vi "1st CMD Operations.vi"(8 "error in (no error)":errorcluster, 10 "Message In":refnum<class "Message.lvclass">, 11 "Node Actor in":refnum<class "Node Actor.lvclass">) -> (0 "error out":errorcluster, 2 "Stop":bool, 3 "Node Actor out":refnum<class "Node Actor.lvclass">)   [LabVIEW 2024, in "Node Actor.lvclass"]
uses:
  Node Actor.lvclass
  Message/Message.lvclass
  Node Actor MSG/Node Actor MSG.lvclass
  Node Actor MSG/Node Actor MSG.lvclass/Node Actor MSG.ctl
  Node Actor MSG/Public Data/Read Node Actor 1st CMD.vi
  Node Actor.lvclass/Node Actor.ctl
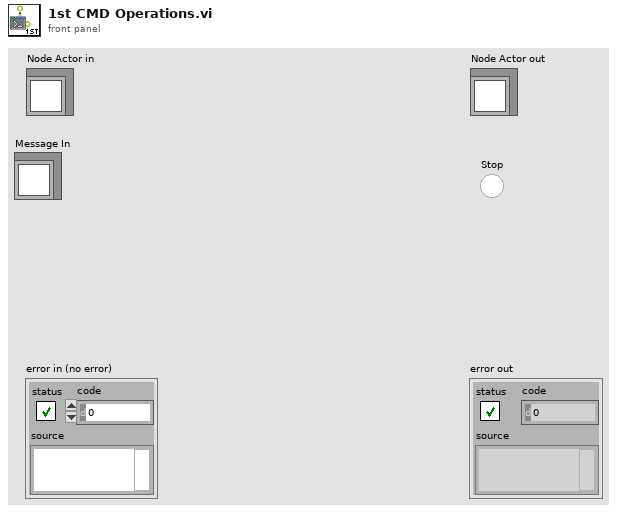
[diagram p1: front panel]
types:
  T1 = typedef "Node Actor 1st CMD.ctl" = enum16{"None", "Message Forward In", "Message Forward Out"}
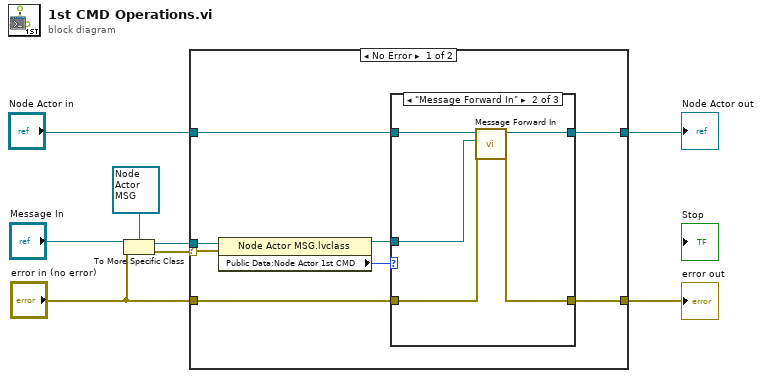
[diagram p0: block diagram]
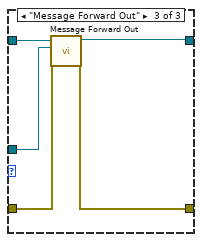
[diagram p3: hidden frame]
diagram:
  n1 = To More Specific Class(target class=refnum<class "Node Actor MSG.lvclass"> refnum ("Node Actor MSG.lvclass"), reference="Message In", error in="error in (no error)") -> (specific class reference=w1:refnum<class "Node Actor MSG.lvclass">, error out=w6:errorcluster)
  n2 = case shown="No Error" w6 {
    selector: w6 -> [w16 _]
    tunnel: "error in (no error)" -> [w10 w30]
    tunnel: [w9 w30] -> w4
    tunnel: [w12 w29] -> w3
    tunnel: "Node Actor in" -> [w14 w29]
    tunnel: w1 -> [w15 _]
    frame No Error {
      n3 = property class="Node Actor MSG.lvclass"(reference=w15, error in=w16) -> (reference out=w11:refnum<class "Node Actor MSG.lvclass">, "Public Data:Node Actor 1st CMD"=w13:T1)  [unwired: 1 out]
      n4 = case shown="\"Message Forward In\"" w13 {
        tunnel: w14 -> [w18 w23 w28]
        tunnel: [w18 w22 w26] -> w12
        tunnel: w11 -> [_ w21 w27]
        tunnel: w10 -> [w17 w20 w25]
        tunnel: [w17 w19 w24] -> w9
        frame "None", Default {
        }
        frame "Message Forward In" {
          n5 = call-dynamic "Message Forward In.vi"("error in (no error)"=w20, "Node Actor MSG In"=w21, "Node Actor in"=w23) -> ("error out"=w19:errorcluster, "Node Actor out"=w22:refnum<class "Node Actor.lvclass">)  [unwired: 7 in]
        }
        frame "Message Forward Out" {
          n6 = call-dynamic "Message Forward Out.vi"("error in (no error)"=w25, "Node Actor MSG In"=w27, "Node Actor in"=w28) -> ("error out"=w24:errorcluster, "Node Actor out"=w26:refnum<class "Node Actor.lvclass">)  [unwired: 7 in]
        }
      }
    }
    frame Error {
    }
  }
  "error out" <- w4
  "Node Actor out" <- w3
